vi "rx streamer recv.vi"(7 "timeout":dbl, 8 "error in (no error)":errorcluster, 9 "md":u64, 10 "buffs":csg[](array[numeric]), 11 "h":u64) -> (0 "error out":errorcluster, 1 "function return":u32(ring), 2 "buffs out":csg[](array[numeric]) format="%.2f", 3 "h 2":u64, 4 "md out":u64, 6 "items_recvd out":u64)   [LabVIEW 2023, in "uhd.lvlib"]
doc: "UHD_API uhd_error uhd_rx_streamer_recv(uhd_rx_streamer_handle h,\n void** buffs,\n size_t samps_per_buff,\n uhd_rx_metadata_handle* md,\n double timeout,\n bool one_packet,\n size_t* items_recvd);"
uses:
  <userlib>/uhd/uhd.lvlib
  <userlib>/uhd/uhd.dll
panel:
  in  "Boolean":bool
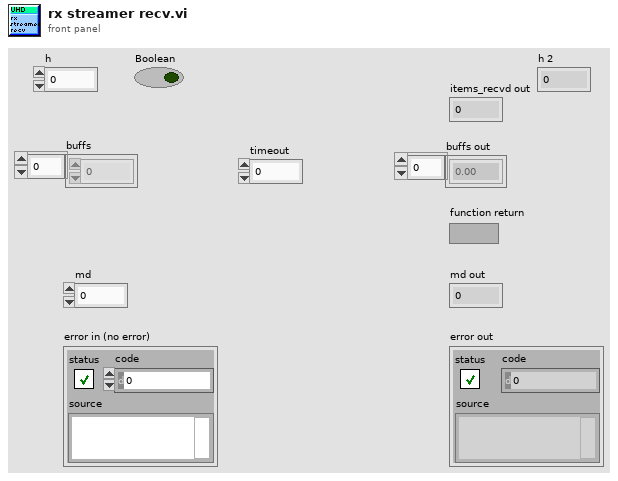
[diagram p1: front panel]
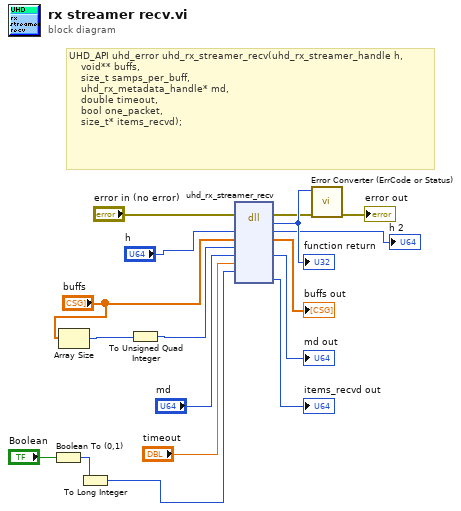
[diagram p0: block diagram]
diagram:
  # "UHD_API uhd_error uhd_rx_streamer_recv(uhd_rx_streamer_handle h,\n    void** buffs,\n    size_t samps_per_buff,\n    uhd_rx_metadata_handle* md,\n    double timeout,\n    bool one_packet,\n    size_t* items_recvd);"
  n1 = Boolean To (0,1)(Boolean="Boolean") -> (0, 1=w4:i16)
  n2 = Array Size(array="buffs") -> (size(s)=w7:i32)
  n3 = To Long Integer(number=w4) -> (32bit integer=w3:i32)
  n4 = To Unsigned Quad Integer(1:w7) -> (0:w6:u64)
  n5 = dll-call lib="C:/Program Files/National Instruments/LabVIEW 2023/user.lib/uhd/uhd.*" fn="uhd_rx_streamer_recv"(error in="error in (no error)", "h"="h", "buffs"="buffs", "samps_per_buff"=w6, "md"="md", "timeout"="timeout", "one_packet"=w3) -> (error out=w10:errorcluster, "return type"=w17:u32, "h"=→"h 2":u64, "buffs"=→"buffs out":csg[], "md"=→"md out":u64, "items_recvd"=→"items_recvd out":u64)  [unwired: 6 in, 1 out]
  "function return" <- w17
  n6 = call <userlib>:"Error Converter (ErrCode or Status).vi"("error in (no error)"=w10, "error code"=w17) -> ("error out"=→"error out":errorcluster)  [unwired: 9 in]
